vi "Draw Vision Mode Overlay 624 Aerial Assist.vi"(9 "Left Cam?":bool, 10 "Vision Mode":T2, 11 "Refnum in":T1) -> (3 "Refnum out":T1)   [LabVIEW 2013]
uses:
  Common Code/Vision Mode.ctl
  <vilib>/vision/Image Controls.llb/IMAQ Image.ctl
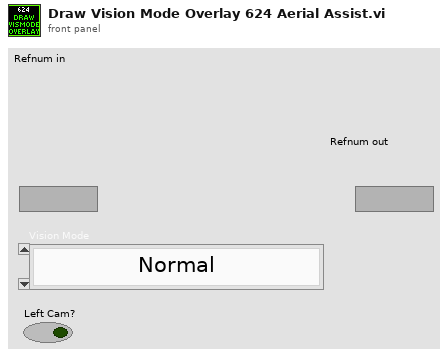
[diagram p1: front panel]
types:
  T1 = typedef "IMAQ Image.ctl" = refnum<image>
  T2 = typedef "Vision Mode.ctl" = enum16{"Normal", "Extreme Left", "Extreme Right"}
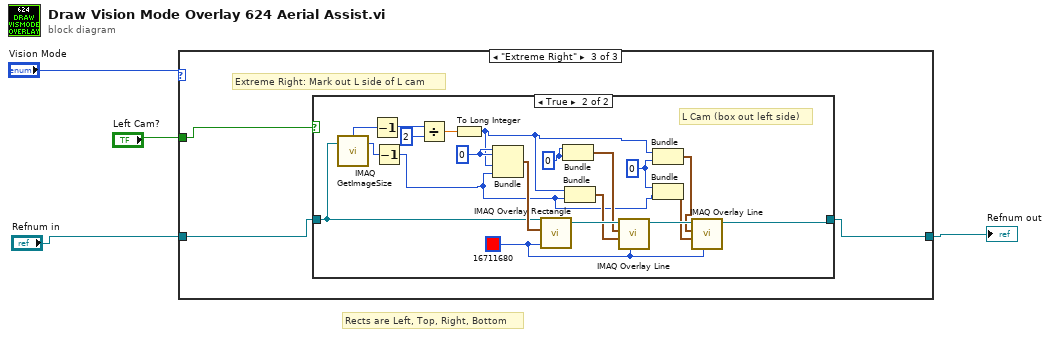
[diagram p0: block diagram]
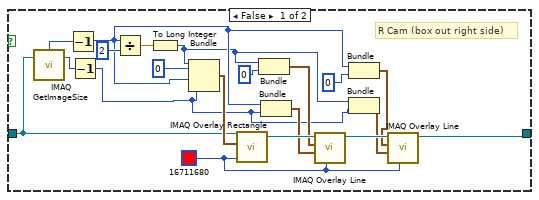
[diagram p4: hidden frame]
diagram:
  # "Rects are Left, Top, Right, Bottom"
  n1 = case shown="\"Extreme Right\"" "Vision Mode" {
    tunnel: "Refnum in" -> [w5 w8 w31]
    tunnel: [w5 w7 w30] -> w2
    tunnel: "Left Cam?" -> [_ w6 w32]
    frame "Normal", Default {
      # "Normal: leave images alone"
    }
    frame "Extreme Left" {
      # "Extreme Left: mark out unused right side of right cam"
      n2 = case shown="True" w6 {
        tunnel: w8 -> [w27 w29]
        tunnel: [w19 w29] -> w7
        frame False {
          w18 = u32 16711680 ("Color")
          # "R Cam (box out right side)"
          n3 = call "IMAQ GetImageSize"("Image"=w27) -> ("Y Resolution"=w25:i32, "X Resolution"=w26:i32)  [unwired: 3 in, 1 out]
          n4 = Decrement(x=w26) -> (x-1=w13:i32)
          n5 = Decrement(x=w25) -> (x-1=w10:i32)
          n6 = Divide(x=w13, y=2) -> (x/y=w23:dbl)
          n7 = To Long Integer(number=w23) -> (32bit integer=w11:i32)
          n8 = Bundle(w11, "y"=0, w13, w10) -> (w28:cluster{i32, "y":i32, i32, i32})  [unwired: 1 in]
          n9 = call "IMAQ Overlay Rectangle"("Color"=w18, "Rectangle"=w28, "Image"=w27) -> ("Image Out"=w21:T1)  [unwired: 7 in, 1 out]
          n10 = Bundle(w11, "y"=0) -> (w16:cluster{i32, "y":i32})  [unwired: 1 in]
          n11 = Bundle(w13, w10) -> (w15:cluster{i32, i32})  [unwired: 1 in]
          n12 = call "IMAQ Overlay Line"("Color"=w18, "End Point"=w15, "Start Point"=w16, "Image"=w21) -> ("Image Out"=w20:T1)  [unwired: 6 in, 1 out]
          n13 = Bundle(w13, "y"=0) -> (w12:cluster{i32, "y":i32})  [unwired: 1 in]
          n14 = Bundle(w11, w10) -> (w9:cluster{i32, i32})  [unwired: 1 in]
          n15 = call "IMAQ Overlay Line"("Color"=w18, "End Point"=w9, "Start Point"=w12, "Image"=w20) -> ("Image Out"=w19:T1)  [unwired: 6 in, 1 out]
        }
        frame True {
          # "L cam"
        }
      }
    }
    frame "Extreme Right" {
      # "Extreme Right: Mark out L side of L cam"
      n16 = case shown="True" w32 {
        tunnel: w31 -> [w33 w52]
        tunnel: [w33 w45] -> w30
        frame False {
          # "L cam"
        }
        frame True {
          w35 = 0 ("y")
          w34 = 0 ("y")
          w44 = u32 16711680 ("Color")
          w38 = 0 ("y")
          # "L Cam (box out left side)"
          n17 = call "IMAQ GetImageSize"("Image"=w52) -> ("Y Resolution"=w50:i32, "X Resolution"=w51:i32)  [unwired: 3 in, 1 out]
          n18 = Decrement(x=w51) -> (x-1=w37:i32)
          n19 = Decrement(x=w50) -> (x-1=w40:i32)
          n20 = Divide(x=w37, y=2) -> (x/y=w48:dbl)
          n21 = To Long Integer(number=w48) -> (32bit integer=w36:i32)
          n22 = Bundle("y"=w38, "y"=w38, w36, w40) -> (w53:cluster{"y":i32, "y":i32, i32, i32})  [unwired: 1 in]
          n23 = call "IMAQ Overlay Rectangle"("Color"=w44, "Rectangle"=w53, "Image"=w52) -> ("Image Out"=w47:T1)  [unwired: 7 in, 1 out]
          n24 = Bundle("y"=w34, "y"=w34) -> (w43:cluster{"y":i32, "y":i32})  [unwired: 1 in]
          n25 = Bundle(w36, w40) -> (w42:cluster{i32, i32})  [unwired: 1 in]
          n26 = call "IMAQ Overlay Line"("Color"=w44, "End Point"=w42, "Start Point"=w43, "Image"=w47) -> ("Image Out"=w46:T1)  [unwired: 6 in, 1 out]
          n27 = Bundle(w36, "y"=w35) -> (w41:cluster{i32, "y":i32})  [unwired: 1 in]
          n28 = Bundle("y"=w35, w40) -> (w39:cluster{"y":i32, i32})  [unwired: 1 in]
          n29 = call "IMAQ Overlay Line"("Color"=w44, "End Point"=w39, "Start Point"=w41, "Image"=w46) -> ("Image Out"=w45:T1)  [unwired: 6 in, 1 out]
        }
      }
    }
  }
  "Refnum out" <- w2
